vi "leso6_temperature.vi"() -> ()   [LabVIEW 2012]
doc: "Программа на LabVIEW. Цифровой термометр.\nВерсия: 0.1\nВерсия LabVIEW: 2012\nОперационная система: MS Windows\nАвтор: Шауэрман Александр. shamrel@yandex.ru\nДата: 28 апреля 2015г.\n\nПрограмма на LabVIEW демонстрирует работу модулей LESO. Визуализирует показание датчика\nтемпературы на стенде LESO6. \nСтатья в интернете: http://www.labfor.ru/articles/labview/leso6_part2"
panel:
  out "Valid":bool
  out "Thermometer":dbl(slide) scale=0.0..40.0
  in  "stop":bool
  out "Bytes Read":u32
  out "Read Data":u8[](array[numeric]) format="%x"
  out "Bytes Written":u32
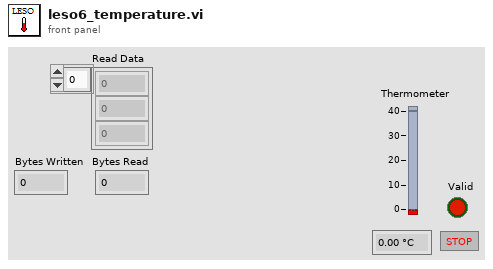
[diagram p1: front panel]
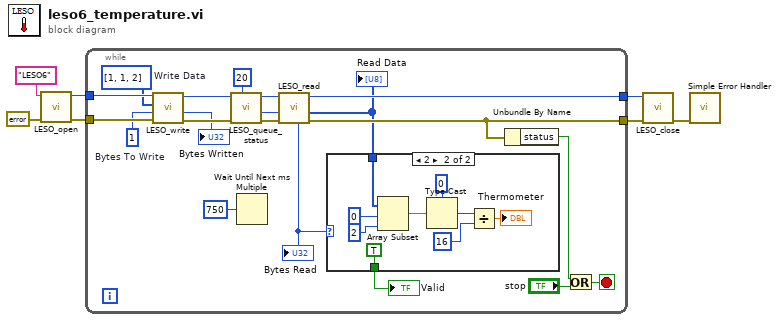
[diagram p0: block diagram]
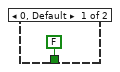
[diagram p2: hidden frame]
diagram:
  n1 = call "LESO_open.vi"("error in"=errorcluster {"status"=FALSE, "code"=0, "source"=""}, "LESO Name"="LESO6") -> ("error out"=w4:errorcluster, "Handle"=w7:u32)  [unwired: 7 in, 1 out]
  n2 = while {
    tunnel: w7 -> [w26]
    tunnel: w4 -> [w25]
    tunnel: [w16] -> w3
    tunnel: [w15] -> w2
    stop <- w13 stop-if-true
    w24 = u8[] [1, 1, 2]  # Write Data
    w23 = u32 1  # Bytes To Write
    n3 = call "LESO_write.vi"("error in"=w25, "Bytes To Write"=w23, "Buffer"=w24, "Handle in"=w26) -> ("error out"=w22:errorcluster, "Bytes Written"=→"Bytes Written":u32, "Handle out"=w27:u32)  [unwired: 4 in, 1 out]
    n4 = call "LESO_queue_status.vi"("milliseconds to wait"=u32 20, "error in"=w22, "Handle in"=w27) -> ("error out"=w19:errorcluster, "Bytes Waiting"=w18:u32, "Handle out"=w20:u32)  [unwired: 5 in, 1 out]
    n5 = Wait Until Next ms Multiple(millisecond multiple=u32 750) -> ()  [unwired: 1 out]
    n6 = call "LESO_read.vi"("error in (no error)"=w19, "Bytes To Read"=w18, "Handle in"=w20) -> ("error out"=w15:errorcluster, "Read Data"=w11:u8[], "Handle Out"=w16:u32, "Bytes Read"=w9:u32)  [unwired: 4 in, 1 out]
    "Bytes Read" <- w9
    "Read Data" <- w11
    n7 = case shown="2" w9 {
      tunnel: w11 -> [_ w37]
      tunnel: [FALSE ("Valid") TRUE ("Valid")] -> w8
      frame 0, Default {
      }
      frame 2 {
        n8 = Array Subset(array=w37, index=0, length=2) -> (w33:u8[])
        n9 = Type Cast(type=i16 0, x=w33) -> (*(type *) &x=w32:i16)
        n10 = Divide(x=w32, y=16) -> (x/y=→"Thermometer":dbl)
      }
    }
    "Valid" <- w8
    n11 = Unbundle By Name(w15) -> ("status"=w12:bool)
    n12 = Or(x=w12, y="stop") -> (x .or. y?=w13:bool)
  }
  n13 = call "LESO_close.vi"("error in (no error)"=w2, "Handle in"=w3) -> ("error out"=w1:errorcluster)  [unwired: 8 in, 1 out]
  n14 = call <vilib>:"Simple Error Handler.vi"("error in (no error)"=w1) -> ()  [unwired: 4 in, 5 out]
